vi "RH_DCPower_Close.vi"(8 "error in (no error)":errorcluster, 9 "Reset?":bool, 10 "channel name":string, 11 "DCPower Session In":refnum<k15>) -> (0 "error out":errorcluster)   [LabVIEW 2023, in "ResourceHandling.lvlib"]
doc: "Reset, disables and closes the resource"
uses:
  ResourceHandling.lvlib
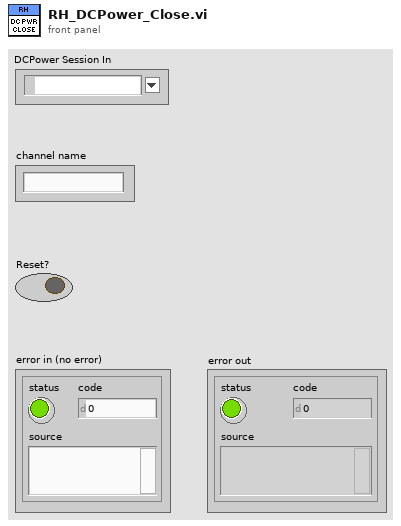
[diagram p1: front panel]
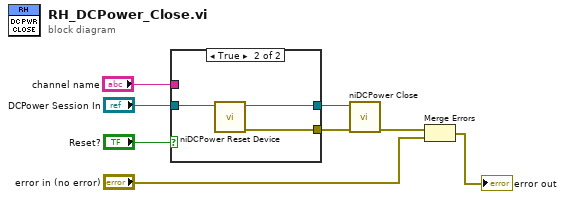
[diagram p0: block diagram]
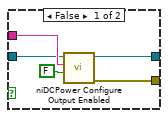
[diagram p2: hidden frame]
diagram:
  n1 = case shown="True" "Reset?" {
    tunnel: [w11 w16] -> w6
    tunnel: [w13 w15] -> w7
    tunnel: "channel name" -> [w10 _]
    tunnel: "DCPower Session In" -> [w9 w14]
    frame False {
      n2 = call <instrlib>:"niDCPower Configure Output Enabled.vi"("output enabled"=FALSE, "channel name"=w10, "instrument handle"=w9) -> ("error out"=w11:errorcluster, "instrument handle out"=w13:refnum<k15>)  [unwired: 7 in]
    }
    frame True {
      n3 = call <instrlib>:"niDCPower Reset Device.vi"("instrument handle"=w14) -> ("error out"=w16:errorcluster, "instrument handle out"=w15:refnum<k15>)  [unwired: 9 in]
    }
  }
  n4 = call <instrlib>:"niDCPower Close.vi"("error in (no error)"=w6, "instrument handle"=w7) -> ("error out"=w8:errorcluster)  [unwired: 9 in]
  n5 = Merge Errors(w8, "error in (no error)") -> (→"error out":errorcluster)
